vi "VCS Activate Analog Position Setpoint.vi"(0 "axis in":cluster{"keyHandle":u32, "nodeId":u16}={"keyHandle"=0, "nodeId"=1}, 7 "analog position setting":T1, 11 "error in (no error)":errorcluster) -> (4 "axis out":cluster{"keyHandle":u32, "nodeId":u16}={"keyHandle"=0, "nodeId"=1}, 15 "error out":errorcluster)   [LabVIEW 2010]
doc: "<B>VCS_ActivateAnalogPositionSetpoint</B> configures the selected analog input for analog position setpoint."
uses:
  Resources/EposCmd.dll
  Resources/EposCmd64.dll
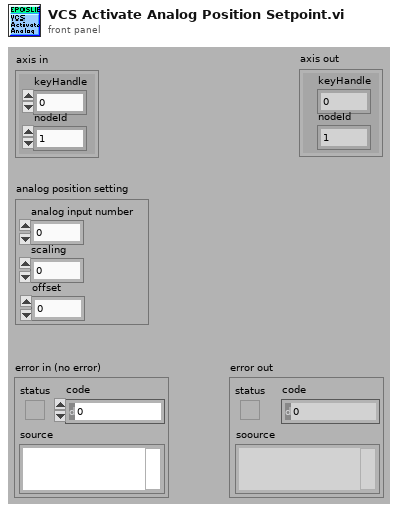
[diagram p1: front panel]
types:
  T1 = cluster{"analog input number":u16, "scaling":sgl, "offset":i32}
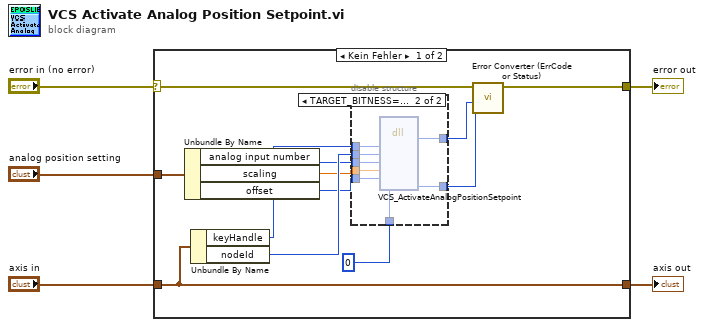
[diagram p0: block diagram]
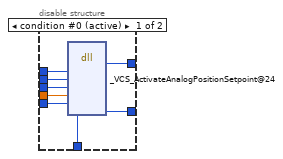
[diagram p2: hidden frame]
diagram:
  n1 = case shown="Kein Fehler" "error in (no error)" {
    selector: "error in (no error)" -> [w15 w34]
    tunnel: "axis in" -> [w17 w35]
    tunnel: [w17 w35] -> w4
    tunnel: [w16 w34] -> w3
    tunnel: "analog position setting" -> [w9 _]
    frame No Error {
      n2 = Unbundle By Name(w9) -> ("analog input number"=w8:u16, "scaling"=w7:sgl, "offset"=w6:i32)
      n3 = Unbundle By Name(w17) -> ("keyHandle"=w14:u32, "nodeId"=w13:u16)
      n4 = disable-structure shown="TARGET_BITNESS==64" {
        disable-tunnel: w14 -> [w25 w33]
        disable-tunnel: w13 -> [w24 w32]
        disable-tunnel: u32 0 ("pErrorCode") -> [w23 w31]
        disable-tunnel: [w22 w30] -> w11
        disable-tunnel: [w21 w29] -> w10
        disable-tunnel: w8 -> [w20 w28]
        disable-tunnel: w7 -> [w19 w27]
        disable-tunnel: w6 -> [w18 w26]
        frame condition #0 (active) {
          n5 = dll-call lib="C:/Sources/LabView/maxon EPOS/Resources/EposCmd.*" fn="_VCS_ActivateAnalogPositionSetpoint@24"("KeyHandle"=w25, "NodeId"=w24, "AnalogInputNumber"=w20, "Scaling"=w19, "Offset"=w18, "pErrorCode"=w23) -> (w21:i32, "pErrorCode"=w22:u32)  [unwired: 8 in, 2 out]
        }
        frame condition #1 {
          n6 = dll-call lib="C:/setup/Resources/EposCmd64.*" fn="VCS_ActivateAnalogPositionSetpoint" ("EposCmd.dll:_VCS_ActivateAnalogPositionSetpoint@24")("KeyHandle"=w33, "NodeId"=w32, "AnalogInputNumber"=w28, "Scaling"=w27, "Offset"=w26, "pErrorCode"=w31) -> ("Rückgabetyp"=w29:i32, "pErrorCode"=w30:u32)  [unwired: 8 in, 2 out]
        }
      }
      n7 = call "Error Converter (ErrCode or Status).vi"("error code"=w11, "return type"=w10, "error in (no error)"=w15) -> ("error out"=w16:errorcluster)  [unwired: 7 in]
    }
    frame Error {
    }
  }
  "error out" <- w3
  "axis out" <- w4
